vi "Generate Random ASCII Character.vi"(3 "ASCII Character Type":T1) -> (0 "ASCII Value":u8 format="%02x", 1 "Random ASCII Character":string)   [LabVIEW 2022 SP3]
doc: "Generates a single random ASCII character, of the requested type.\n\nTypes:\n1. Lowercase Letter: ASCII 0x41 to 0x5A\n2. Uppercase Letter: ASCII 0x61 to 0x7A\n3. Digit: ASCII 0x30 to 0x39\n4. Alphanumeric = Lowercase Letter, Uppercase Letter or Digit\n5. Printable Character: ASCII 0x20 to 0x7F\n6. Any ASCII Character: ASCII 0x00 to 0xFF\n\nASCII table: http://www.asciitable.com/\n\nPerformance: This VI is inlined to increase performance"
uses:
  ASCII Character Type.ctl
  <vilib>/numeric/Random Number (Range) U64.vi
  <vilib>/numeric/sub_Random U32.vi
panel:
  # "Development\ncontrols/indicators useful for development and testing, but which are not outputs of the VI"
  # "Input\nInputs to the VI"
  # "Output\nOutputs of the VI"
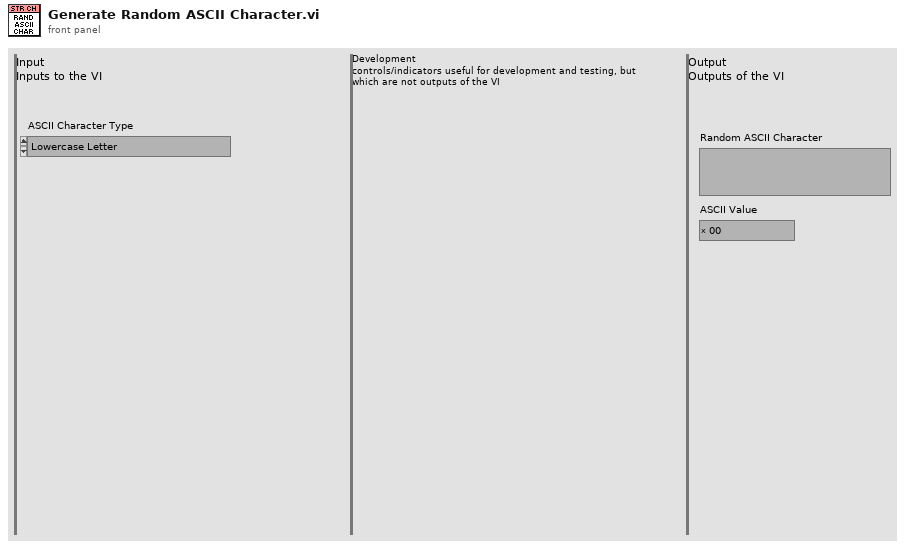
[diagram p1: front panel]
types:
  T1 = typedef "ASCII Character Type.ctl" = enum16{"Lowercase Letter", "Uppercase Letter", "Digit", "Alphanumeric", "Printable Character", "Any ASCII Character [0x00 to 0xFF]"}
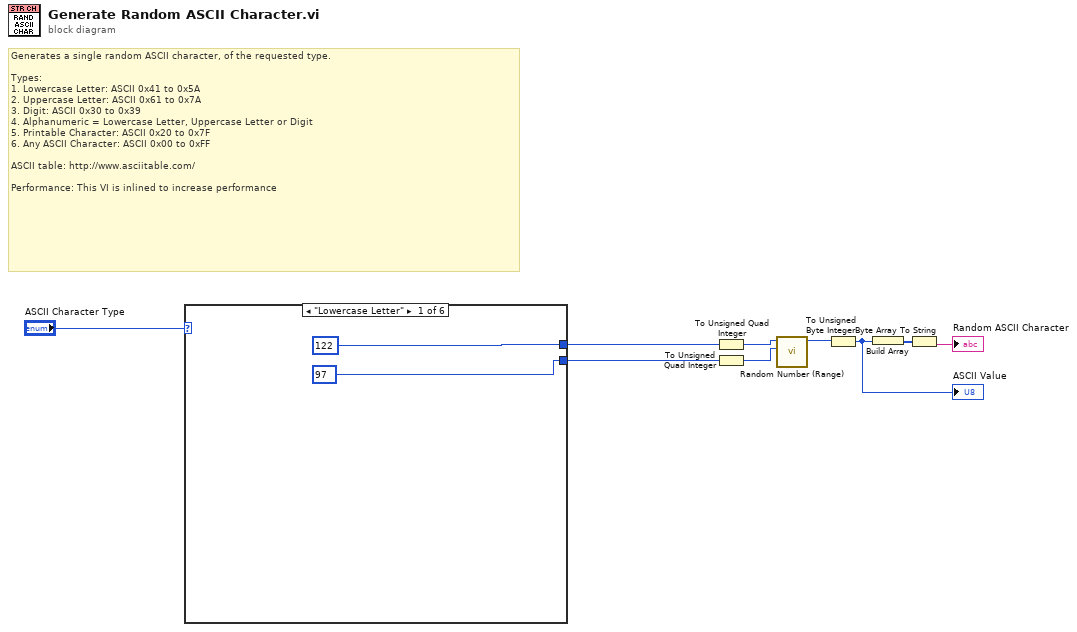
[diagram p0: block diagram]
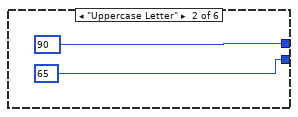
[diagram p2: hidden frame]
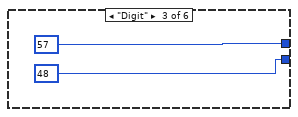
[diagram p3: hidden frame]
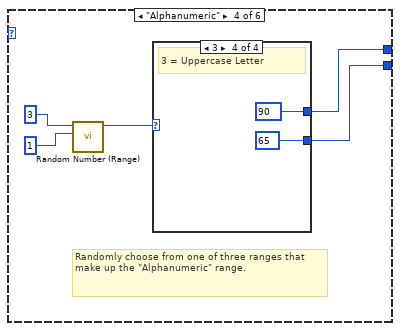
[diagram p4: hidden frame]
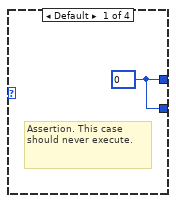
[diagram p5: hidden frame]
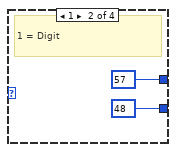
[diagram p6: hidden frame]
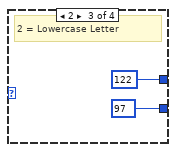
[diagram p7: hidden frame]
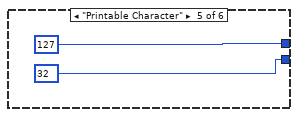
[diagram p8: hidden frame]
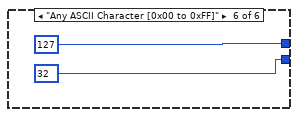
[diagram p9: hidden frame]
diagram:
  # "Generates a single random ASCII character, of the requested type.\n\nTypes:\n1. Lowercase Letter: ASCII 0x41 to 0x5A\n2. Uppercase Letter: ASCII 0x61 to 0x7A\n3. Digit: ASCII 0x30 to 0x39\n4. Alphanumeric = Lowercase Letter, Uppercase Letter or Digit\n5. Printable Character: ASCII 0x20 to 0x7F\n6. Any ASCII Character: ASCII 0x00 to 0xFF\n\nASCII table: http://www.asciitable.com/\n\nPerformance: This VI is inlined to increase performance"
  n1 = case shown="\"Lowercase Letter\"" "ASCII Character Type" {
    tunnel: [u8 97 u8 65 u8 48 w19 u8 32 u8 32] -> w8
    tunnel: [u8 122 u8 90 u8 57 w20 u8 127 u8 127] -> w7
    frame "Lowercase Letter" {
    }
    frame "Uppercase Letter" {
    }
    frame "Digit" {
    }
    frame "Alphanumeric" {
      # "Randomly choose from one of three ranges that make up the \"Alphanumeric\" range."
      n2 = call-poly <vilib>:"Random Number (Range).vi"("lower bound (0)"=u64 1 ("Low"), "upper bound (100)"=u64 3 ("High")) -> ("number"=w16:u64)  [unwired: 9 in]
      n3 = case shown="3" w16 {
        tunnel: [w21 u8 57 u8 122 u8 90] -> w20
        tunnel: [w21 u8 48 u8 97 u8 65] -> w19
        frame Default {
          w21 = u8 0
          # "Assertion. This case should never execute."
        }
        frame 1 {
          # "1 = Digit"
        }
        frame 2 {
          # "2 = Lowercase Letter"
        }
        frame 3 {
          # "3 = Uppercase Letter"
        }
      }
    }
    frame "Printable Character" {
    }
    frame "Any ASCII Character [0x00 to 0xFF]" {
    }
  }
  n4 = To Unsigned Quad Integer(1:w7) -> (0:w3:u64)
  n5 = To Unsigned Quad Integer(1:w8) -> (0:w2:u64)
  n6 = call-poly <vilib>:"Random Number (Range).vi"("lower bound (0)"=w2, "upper bound (100)"=w3) -> ("number"=w1:u64)  [unwired: 9 in]
  n7 = To Unsigned Byte Integer(number=w1) -> (unsigned 8bit integer=w5:u8)
  "ASCII Value" <- w5
  n8 = Build Array(w5) -> (w9:u8[])
  n9 = Byte Array To String(unsigned byte array=w9) -> (string=→"Random ASCII Character":string)
